vi "Log Error.vi"(10 "error in (no error)":errorcluster, 11 "DAQ Actor in":refnum<class "DAQ Actor.lvclass">) -> (0 "error out":errorcluster, 2 "Error Count":u32, 3 "DAQ Actor out":refnum<class "DAQ Actor.lvclass">)   [LabVIEW 2018, in "Data Acquisition.lvlib" / "DAQ Actor.lvclass"]
uses:
  DAQ Actor.lvclass
  DAQ Actor.lvclass/DAQ Actor.ctl
  Cfg Grandmaster/Class Cfg Grandmaster/Cfg Grandmaster.lvclass
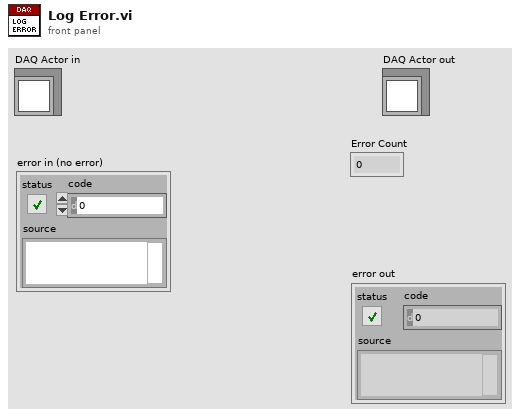
[diagram p1: front panel]
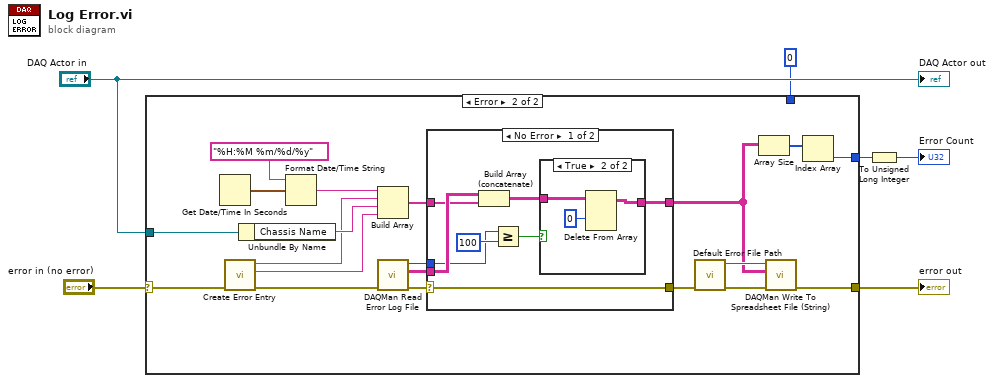
[diagram p0: block diagram]
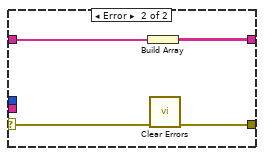
[diagram p4: hidden frame]
diagram:
  n1 = case shown="Error" "error in (no error)" {
    selector: "error in (no error)" -> [w8 w12]
    tunnel: [w8 w24] -> w6
    tunnel: "DAQ Actor in" -> [_ w23]
    tunnel: [w7 w18] -> w2
    tunnel: 0 -> [w7 _]
    frame No Error {
    }
    frame Error {
      n2 = Get Date/Time In Seconds() -> (seconds since 1Jan1904=w27:timestamp)
      n3 = call "Create Error Entry.vi"("error in (no error)"=w12) -> ("error out"=w11:errorcluster, "Description"=w9:string, "Code"=w10:string)  [unwired: 8 in]
      n4 = Unbundle By Name(w23) -> ("Chassis Name"=w25:string)
      n5 = Format Date/Time String(time format string (%c)="%H:%M %m/%d/%y", seconds (now)=w27) -> (date/time string=w26:string)  [unwired: 1 in]
      n6 = Build Array(w26, w10, w25, w9) -> (w22:string[])
      n7 = call "DAQMan Read Error Log File.vi"("error in (no error)"=w11) -> ("error out"=w17:errorcluster, "all rows"=w16:string[][], "Number of Rows"=w15:u32)  [unwired: 8 in]
      n8 = case shown="No Error" w17 {
        selector: w17 -> [w30 w42]
        tunnel: w16 -> [w36 _]
        tunnel: w22 -> [w35 w44]
        tunnel: [w31 w43] -> w19
        tunnel: [w30 w41] -> w14
        tunnel: w15 -> [w29 _]
        frame No Error {
          n9 = Build Array (concatenate)(w36, w35) -> (w34:string[][])
          n10 = Greater Or Equal?(x=w29, y=u32 100) -> (x >= y?=w32:bool)
          n11 = case shown="True" w32 {
            tunnel: [w37 w39] -> w31
            tunnel: w34 -> [w37 w38]
            frame False {
            }
            frame True {
              n12 = Delete From Array(array=w38, index (row)=0) -> (array with subset deleted=w39:string[][])  [unwired: 2 in, 1 out]
            }
          }
        }
        frame Error {
          n13 = Build Array(w44) -> (w43:string[][])
          n14 = call <vilib>:"Clear Errors.vi"("error in (no error)"=w42) -> ("error out"=w41:errorcluster)  [unwired: 5 in, 1 out]
        }
      }
      n15 = call "Default Error File Path.vi"("error in (no error)"=w14) -> ("error out"=w13:errorcluster, "Default Path"=w21:path)  [unwired: 9 in]
      n16 = Array Size(array=w19) -> (size(s)=w20:i32[])
      n17 = call "DAQMan Write To Spreadsheet File (String).vi"("error in"=w13, "2D data"=w19, "file path (dialog if empty)"=w21) -> ("error out"=w24:errorcluster)  [unwired: 7 in, 1 out]
      n18 = Index Array(array=w20) -> (element=w18:i32)  [unwired: 1 in]
    }
  }
  "error out" <- w6
  n19 = To Unsigned Long Integer(number=w2) -> (unsigned 32bit integer=→"Error Count":u32)
  "DAQ Actor out" <- "DAQ Actor in"
